vi "VI-Find Project Item (LVClass).vi"(0 "LVClassLibrary Refnum":refnum<vi>, 5 "Type":string, 7 "Name":string, 11 "error in (no error)":errorcluster) -> (4 "reference out":refnum<vi>, 6 "ProjectItem":refnum<vi>, 15 "error out":errorcluster)   [LabVIEW 2020]
panel:
  out "Found":bool
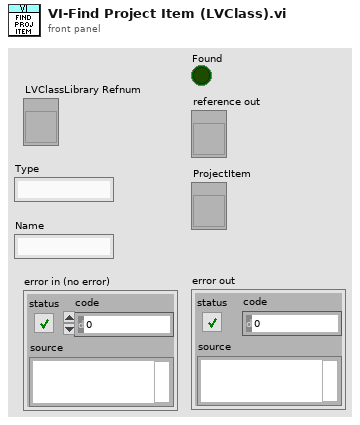
[diagram p1: front panel]
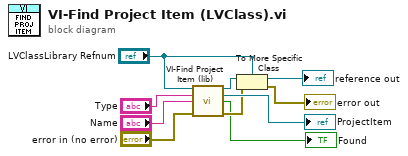
[diagram p0: block diagram]
diagram:
  n1 = call "VI-Find Project Item (lib).vi"("Library Refnum"="LVClassLibrary Refnum", "Type"="Type", "Name"="Name", "error in (no error)"="error in (no error)") -> ("reference out"=w6:refnum<vi>, "ProjectItem"=→"ProjectItem":refnum<vi>, "Found"=→"Found":bool, "error out"=w3:errorcluster)  [unwired: 8 in]
  n2 = To More Specific Class(target class="LVClassLibrary Refnum", reference=w6, error in=w3) -> (specific class reference=→"reference out":refnum<vi>, error out=→"error out":errorcluster)
